vi "LV86_Morph_AutoMedian.vi"(2 "Connectivity":enum16{"4", "6", "8"}(ring), 3 "Image in":T1 {"Dialogs" format="%.0b"}) -> (1 "Image out":T1 {"Dialogs" format="%.0b"})   [LabVIEW 2024]
doc: "This VI uses dual combinations of openings and closings. It generates simpler particles that have fewer details."
uses:
  <userlib>/ImageProcessing/QTLIB_2595_LV86/QT_Image.ctl
panel:
  out "Auto median":picture caption="new picture"
  out "Initial Image":picture caption="new picture"
  # "This VI uses dual combinations of openings and closings.  \nIt generates simpler particles that have fewer details."
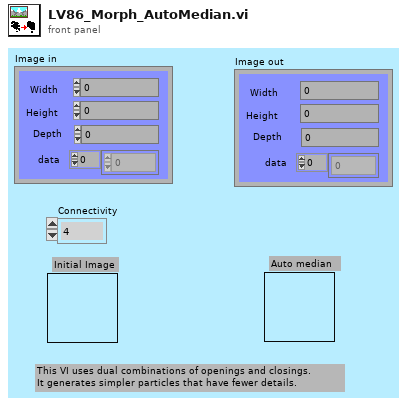
[diagram p1: front panel]
types:
  T1 = typedef "QT_Image.ctl" = cluster{"Width":i32, "Height":i32, "Depth":i32, "data":u8[], "Compressed data":u8[], "Color table":u32[], "Duration":i32, "Options":i32, "Timestamp":i32, "ID":i32, "Reserved":i32, "Dialogs":u32}
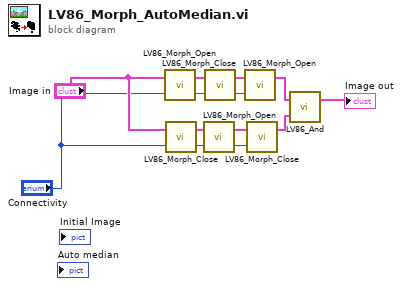
[diagram p0: block diagram]
diagram:
  n1 = call <userlib>:"LV86_Morph_Open.vi"("Connectivity"="Connectivity", "Image in"="Image in") -> ("Image out"=w9:T1)  [unwired: 1 out]
  n2 = call <userlib>:"LV86_Morph_Close.vi"("Connectivity"="Connectivity", "Image in"="Image in") -> ("Image out"=w7:T1)  [unwired: 1 out]
  n3 = call <userlib>:"LV86_Morph_Open.vi"("Connectivity"="Connectivity", "Image in"=w7) -> ("Image out"=w6:T1)  [unwired: 1 out]
  n4 = call <userlib>:"LV86_Morph_Close.vi"("Connectivity"="Connectivity", "Image in"=w9) -> ("Image out"=w8:T1)  [unwired: 1 out]
  n5 = call <userlib>:"LV86_Morph_Open.vi"("Connectivity"="Connectivity", "Image in"=w8) -> ("Image out"=w4:T1)  [unwired: 1 out]
  n6 = call <userlib>:"LV86_Morph_Close.vi"("Connectivity"="Connectivity", "Image in"=w6) -> ("Image out"=w5:T1)  [unwired: 1 out]
  n7 = call <userlib>:"LV86_And.vi"("Image 2"=w5, "Image"=w4) -> ("Image Out"=→"Image out":T1)  [unwired: 1 in]
